vi "calcForceError.vi"(8 "error in (no error)":errorcluster, 11 "Model in":refnum<class "Model.lvclass">) -> (0 "error out":errorcluster, 3 "Model out":refnum<class "Model.lvclass">)   [LabVIEW 2013, in "Model.lvclass"]
uses:
  Model.lvclass
  Typedefs/ControllerData.ctl
  Typedefs/ForceDemand.ctl
  Model.lvclass/Model.ctl
  <userlib>/Common/Devices/ForceSensorCalculator/ForceSensorCalculator/ForceSensorCalculator.lvclass/ForceSensorCalculator.ctl
  ApplicationElements/SystemController/SystemController.lvclass/SystemController.ctl
  UserEvents/UserEvents.lvclass/UserEvents.ctl
  ApplicationElements/Log/TestDataLog/TestDataLog.lvclass/TestDataLog.ctl
  ApplicationElements/SystemController/SystemController.lvclass
  <userlib>/Common/Devices/ForceSensorCalculator/ForceSensorCalculator/ForceSensorCalculator.lvclass
  Typedefs/M2AADTTypedefs.lvlib
  UserEvents/UserEvents.lvclass
  ApplicationElements/Log/TestDataLog/TestDataLog.lvclass
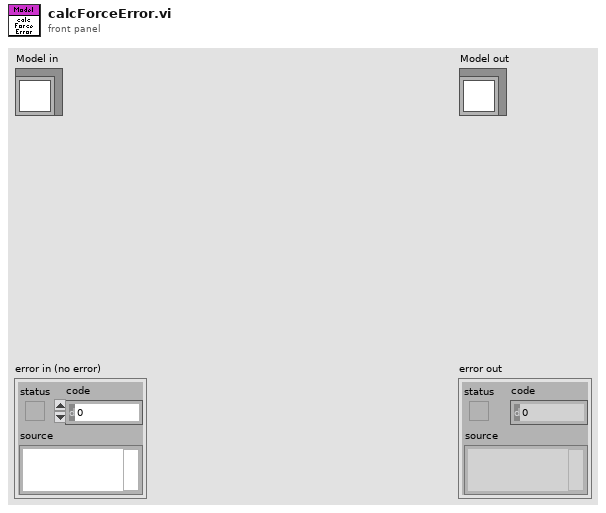
[diagram p1: front panel]
types:
  T1 = typedef "M2AADTTypedefs.lvlib/ControllerData.ctl" = cluster{"Force Demand":T2, "Force Error":T2}
  T2 = typedef "M2AADTTypedefs.lvlib/ForceDemand.ctl" = dbl[unit]
  T3 = typedef "M2AADTTypedefs.lvlib/PubDataEvents.ctl" = cluster{"State":refnum<user-event>, "ErrorCode":refnum<user-event>, "OutputData":refnum<user-event>, "InputData":refnum<user-event>, "ControllerData":refnum<user-event>, "TestStatus":refnum<user-event>, "LogPath":refnum<user-event>, "StiffnessData":refnum<user-event>}
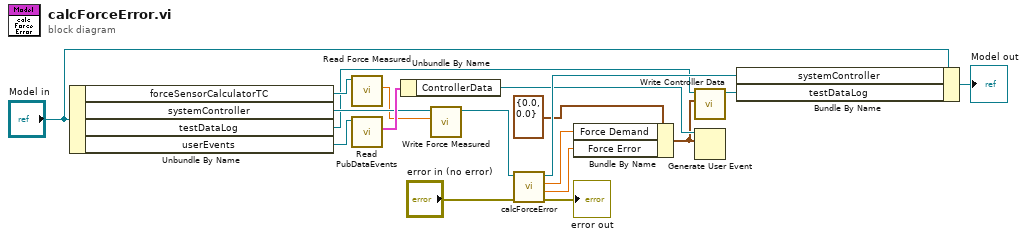
[diagram p0: block diagram]
diagram:
  n1 = Unbundle By Name("Model in") -> ("forceSensorCalculatorTC"=w15:refnum<class "ForceSensorCalculatorTC.lvclass">, "systemController"=w6:refnum<class "SystemController.lvclass">, "testDataLog"=w3:refnum<class "TestDataLog.lvclass">, "userEvents"=w7:refnum<class "UserEvents.lvclass">)
  n2 = call <userlib>:"Read Force Measured.vi"("ForceSensor in"=w15) -> ("Force Demand"=w4:dbl[unit])  [unwired: 9 in, 1 out]
  n3 = call "Read PubDataEvents.vi"("UserEvents in"=w7) -> ("PubDataEvents"=w9:T3)  [unwired: 9 in, 1 out]
  n4 = Unbundle By Name(w9) -> ("ControllerData"=w8:refnum<user-event>)
  n5 = call "Write Force Measured.vi"("Force Demand"=w4, "SystemController in"=w6) -> ("SystemController out"=w5:refnum<class "SystemController.lvclass">)  [unwired: 9 in]
  n6 = call "calcForceError.vi"("error in (no error)"="error in (no error)", "SystemController in"=w5) -> ("error out"=→"error out":errorcluster, "Force Error"=w11:T2, "Force Demand"=w10:T2, "SystemController out"=w16:refnum<class "SystemController.lvclass">)  [unwired: 6 in]
  n7 = Bundle By Name(cluster=T1 {"Force Demand"=0.0, "Force Error"=0.0} ("event data"), "Force Demand"=w10, "Force Error"=w11) -> (w2:T1)
  n8 = call "Write Controller Data.vi"("Controller Data"=w2, "Logger in"=w3) -> ("Logger out"=w1:refnum<class "TestDataLog.lvclass">)  [unwired: 9 in]
  n9 = Generate User Event(user event=w8, event data cluster=w2) -> ()  [unwired: 2 in, 2 out]
  n10 = Bundle By Name(cluster="Model in", "systemController"=w16, "testDataLog"=w1) -> (→"Model out":refnum<class "Model.lvclass">)
